vi "16T_Queue_Commands.vi"(1 "16 T Magnet control":T2={"Clamp"=FALSE, "Switch Heater"=FALSE, "Go to Zero"=FALSE, "Go to Set"=FALSE, "Go to Hold"=FALSE, "Setpoint (T)"=3.4572, "Rate (T/min)"=0.0, "Set Rate"=FALSE} {"Rate (T/min)" format="%6_5f"; "Setpoint (T)" format="%#4_5f"}, 3 "16T Queue":refnum<queue>) -> (0 "New Status":T2={"Clamp"=FALSE, "Switch Heater"=FALSE, "Go to Zero"=FALSE, "Go to Set"=FALSE, "Go to Hold"=FALSE, "Setpoint (T)"=3.4572, "Rate (T/min)"=0.0, "Set Rate"=FALSE} {"Rate (T/min)" format="%6_5f"; "Setpoint (T)" format="%#4_5f"})   [LabVIEW 2018]
uses:
  S16/16T_Control.ctl
panel:
  out "x = y?":T1
  # "20 T"
  # "20 T"
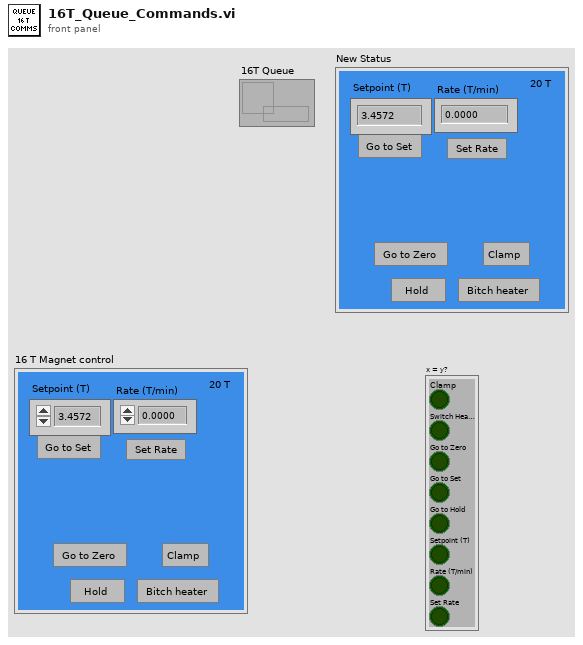
[diagram p1: front panel]
types:
  T1 = cluster{"Clamp":bool, "Switch Heater":bool, "Go to Zero":bool, "Go to Set":bool, "Go to Hold":bool, "Setpoint (T)":bool, "Rate (T/min)":bool, "Set Rate":bool}
  T2 = typedef "16T_Control.ctl" = cluster{"Clamp":bool, "Switch Heater":bool, "Go to Zero":bool, "Go to Set":bool, "Go to Hold":bool, "Setpoint (T)":dbl, "Rate (T/min)":dbl, "Set Rate":bool}
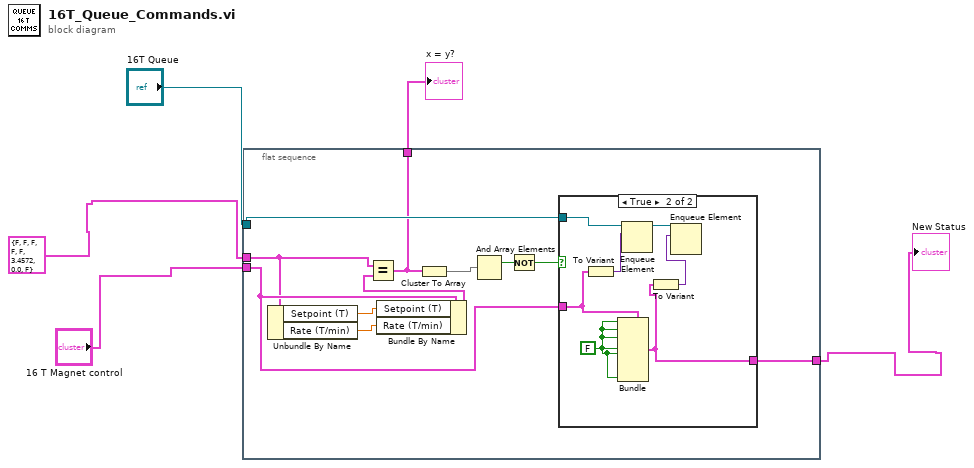
[diagram p0: block diagram]
diagram:
  n1 = flat-sequence {
    tunnel: "16T Queue" -> [w16]
    tunnel: "16 T Magnet control" -> [w11]
    tunnel: T2 {"Clamp"=FALSE, "Switch Heater"=FALSE, "Go to Zero"=FALSE, "Go to Set"=FALSE, "Go to Hold"=FALSE, "Setpoint (T)"=3.4572, "Rate (T/min)"=0.0, "Set Rate"=FALSE} ("Last Status") -> [w9]
    tunnel: [w12] -> w2
    tunnel: [w6] -> w1
    frame #0 {
      n2 = Unbundle By Name(w9) -> ("Setpoint (T)"=w8:dbl, "Rate (T/min)"=w7:dbl)
      n3 = Bundle By Name(cluster=w11, "Setpoint (T)"=w8, "Rate (T/min)"=w7) -> (w10:T2)
      n4 = Equal?(x=w9, y=w10) -> (x = y?=w6:T1)
      n5 = Cluster To Array(cluster=w6) -> (array=w15:bool[])
      n6 = And Array Elements(Boolean array=w15) -> (logical AND=w14:bool)
      n7 = Not(x=w14) -> (.not. x?=w13:bool)
      n8 = case shown="True" w13 {
        tunnel: w16 -> [_ w24]
        tunnel: w11 -> [w17 w20]
        tunnel: [w17 w19] -> w12
        frame False {
        }
        frame True {
          w18 = FALSE
          n9 = To Variant(anything=w20) -> (Variant=w23:variant)
          n10 = Bundle(cluster=w20, "Clamp"=w18, "Switch Heater"=w18, "Go to Zero"=w18, "Go to Set"=w18, "Go to Hold"=w18, "Set Rate"=w18) -> (w19:T2)  [unwired: 2 in]
          n11 = Enqueue Element(queue=w24, element=w23) -> (queue out=w22:refnum<queue>)  [unwired: 2 in, 2 out]
          n12 = To Variant(anything=w19) -> (Variant=w21:variant)
          n13 = Enqueue Element(queue=w22, element=w21) -> ()  [unwired: 2 in, 3 out]
        }
      }
    }
  }
  "New Status" <- w2
  "x = y?" <- w1
